vi "My Standard Deviation and Variance.vi"(10 "Array - Numeric":dbl[](array[numeric])) -> (0 "Mean":dbl, 1 "Standard Deviation":dbl, 2 "Variance":dbl, 3 "Relative Standard Deviation":dbl)   [LabVIEW 2016]
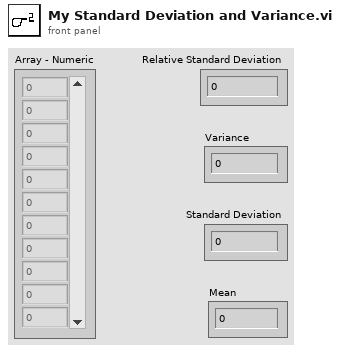
[diagram p1: front panel]
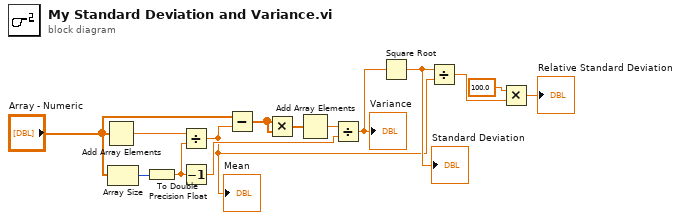
[diagram p0: block diagram]
diagram:
  n1 = Add Array Elements(numeric array="Array - Numeric") -> (sum=w14:dbl)
  n2 = Array Size(array="Array - Numeric") -> (size(s)=w13:i32)
  n3 = To Double Precision Float(number=w13) -> (double precision float=w12:dbl)
  n4 = Divide(x=w14, y=w12) -> (x/y=w4:dbl)
  "Mean" <- w4
  n5 = Decrement(x=w12) -> (x-1=w7:dbl)
  n6 = Subtract(x="Array - Numeric", y=w4) -> (x-y=w10:dbl[])
  n7 = Multiply(x=w10, y=w10) -> (x*y=w9:dbl[])
  n8 = Add Array Elements(numeric array=w9) -> (sum=w8:dbl)
  n9 = Divide(x=w8, y=w7) -> (x/y=w6:dbl)
  "Variance" <- w6
  n10 = Square Root(x=w6) -> (sqrt(x)=w5:dbl)
  "Standard Deviation" <- w5
  n11 = Divide(x=w5, y=w4) -> (x/y=w2:dbl)
  n12 = Multiply(x=100.0, y=w2) -> (x*y=→"Relative Standard Deviation":dbl)
